vi "Read last position.vi"(8 "error in (no error)":errorcluster, 11 "_delayStageBase in":refnum<class "_delayStageBase.lvclass">) -> (0 "error out":errorcluster, 2 "last position":dbl, 3 "_delayStageBase out":refnum<class "_delayStageBase.lvclass">)   [LabVIEW 2019, in "_delayStageBase.lvclass"]
uses:
  _delayStageBase.lvclass
  _delayStageBase.lvclass/_delayStageBase.ctl
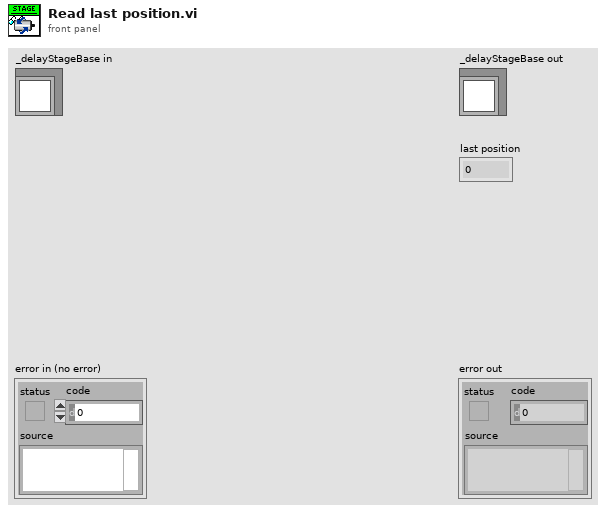
[diagram p1: front panel]
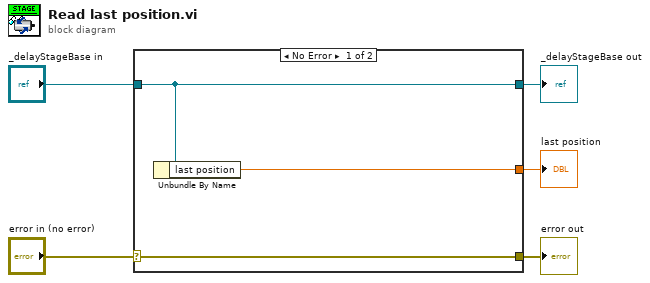
[diagram p0: block diagram]
diagram:
  n1 = case shown="No Error" "error in (no error)" {
    selector: "error in (no error)" -> [w8 w9]
    tunnel: [w8 w9] -> w4
    tunnel: [w7 w10] -> w2
    tunnel: "_delayStageBase in" -> [w7 w10]
    tunnel: [w6 _] -> w1
    frame No Error {
      n2 = Unbundle By Name(w7) -> ("last position"=w6:dbl)
    }
    frame Error {
    }
  }
  "error out" <- w4
  "_delayStageBase out" <- w2
  "last position" <- w1
